vi "test_error_handler.vi"() -> ()   [LabVIEW 2020]
uses:
  <vilib>/Utility/error.llb/Error Cluster From Error Code.vi
  <vilib>/ErrorRing/Error Ring.xnode
panel:
  out "source":string
  out "Array":dbl[](array[numeric])
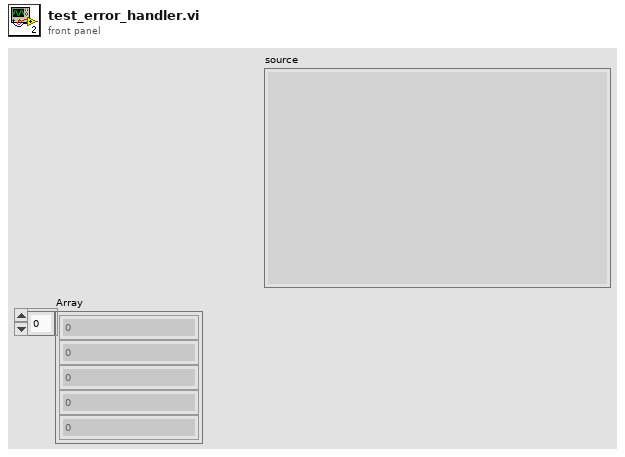
[diagram p1: front panel]
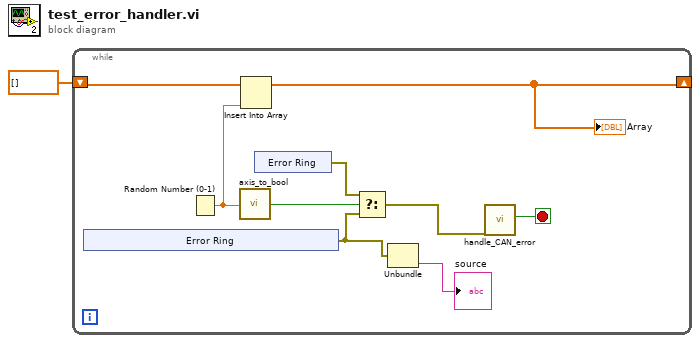
[diagram p0: block diagram]
diagram:
  n1 = while {
    shift-right: [w5] -> _
    shift-left: dbl[] [] -> [w7]
    stop <- w4 stop-if-true
    n2 = xnode "Error Ring"() -> ("error out"=w3:errorcluster)
    n3 = Random Number (0-1)() -> (number: 0 to 1=w6:dbl)
    n4 = call "axis_to_bool.vi"("in"=w6) -> ("out"=w10:bool)
    n5 = Insert Into Array(array=w7, new element=w6) -> (w5:dbl[])  [unwired: 1 in]
    "Array" <- w5
    n6 = xnode "Error Ring"() -> ("error out"=w9:errorcluster)
    n7 = Select(t=w9, s=w10, f=w3) -> (s? t:f=w8:errorcluster)
    n8 = Unbundle(w3) -> ("source"=→"source":string)  [unwired: 2 out]
    n9 = call "handle_CAN_error.vi"("error in (no error)"=w8) -> ("stop"=w4:bool)  [unwired: 9 in, 1 out]
  }
